vi "Hit Detect.vi"(7 "Visible only? [T]":bool=TRUE, 8 "error in (no error)":errorcluster, 10 "Coords":T1, 11 "IObject in":refnum<class "IObject.lvclass">) -> (0 "error out":errorcluster, 1 "Hit?":bool, 2 "In Object":string[](array[string]), 3 "IObject out":refnum<class "IObject.lvclass">)   [LabVIEW 2021, in "IObject.lvclass"]
uses:
  IObject.lvclass
  <vilib>/Utility/miscctls.llb/LVPoint32TypeDef.ctl
  IObject.lvclass/IObject.ctl
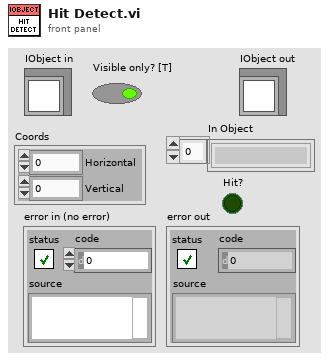
[diagram p1: front panel]
types:
  T1 = typedef "LVPoint32TypeDef.ctl" = cluster{"Horizontal":i32, "Vertical":i32}
  T2 = typedef "LVRectTypeDef.ctl" = cluster{"Left":i16, "Top":i16, "Right":i16, "Bottom":i16}
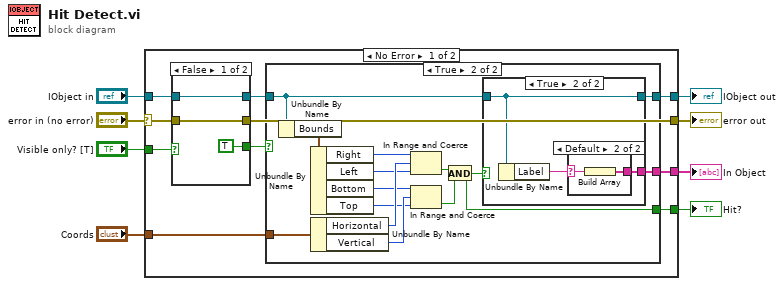
[diagram p0: block diagram]
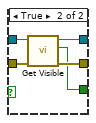
[diagram p5: hidden frame]
diagram:
  n1 = case shown="No Error" "error in (no error)" {
    selector: "error in (no error)" -> [w18 w49]
    tunnel: [w17 w49] -> w7
    tunnel: [w12 w48] -> w5
    tunnel: "IObject in" -> [w16 w48]
    tunnel: "Coords" -> [w15 _]
    tunnel: "Visible only? [T]" -> [w13 _]
    tunnel: [w10 _] -> w2
    tunnel: [w9 _] -> w1
    frame No Error {
      n2 = case shown="False" w13 {
        tunnel: w18 -> [w41 w47]
        tunnel: [w41 w46] -> w17
        tunnel: w16 -> [w42 w45]
        tunnel: [w42 w44] -> w14
        tunnel: [TRUE ("Visible?") w43] -> w11
        frame False {
        }
        frame True {
          n3 = call-dynamic "Get Visible.vi"("error in (no error)"=w47, "IObject in"=w45) -> ("error out"=w46:errorcluster, "Visible?"=w43:bool, "IObject out"=w44:refnum<class "IObject.lvclass">)  [unwired: 6 in, 1 out]
        }
      }
      n4 = case shown="True" w11 {
        tunnel: w15 -> [_ w28]
        tunnel: w14 -> [w19 w23]
        tunnel: [w19 w22] -> w12
        tunnel: [_ w21] -> w10
        tunnel: [_ w20] -> w9
        frame False {
        }
        frame True {
          n5 = Unbundle By Name(w23) -> ("Bounds"=w27:T2)
          n6 = Unbundle By Name(w27) -> ("Right"=w26:i16, "Left"=w31:i16, "Bottom"=w25:i16, "Top"=w24:i16)
          n7 = Unbundle By Name(w28) -> ("Horizontal"=w33:i32, "Vertical"=w32:i32)
          n8 = In Range and Coerce(upper limit=w26, x=w33, lower limit=w31) -> (In Range?=w30:bool)  [unwired: 1 out]
          n9 = In Range and Coerce(upper limit=w25, x=w32, lower limit=w24) -> (In Range?=w29:bool)  [unwired: 1 out]
          n10 = And(x=w30, y=w29) -> (x .and. y?=w20:bool)
          n11 = case shown="True" w20 {
            tunnel: w23 -> [w34 w37]
            tunnel: [w34 w37] -> w22
            tunnel: [_ w36] -> w21
            frame False {
            }
            frame True {
              n12 = Unbundle By Name(w37) -> ("Label"=w35:string)
              n13 = case shown="Default" w35 {
                selector: w35 -> [_ w38]
                tunnel: [_ w39] -> w36
                frame "" {
                }
                frame Default {
                  n14 = Build Array(w38) -> (w39:string[])
                }
              }
            }
          }
        }
      }
    }
    frame Error {
    }
  }
  "error out" <- w7
  "IObject out" <- w5
  "In Object" <- w2
  "Hit?" <- w1
